vi "Sim_Main.vi"() -> ()   [LabVIEW 2009]
panel:
  in  "on or off":bool=TRUE
  in  "Right Thrust 2":dbl
  in  "Left Thrust 2":dbl
  out "Waveform Graph":cluster{dbl, "Delta t":dbl, "elements":dbl[]}(graph)
  in  "Inertia":dbl=10.0
  in  "max queue size (-1, unlimited)":i32=10
  out "XY Graph":T1(graph)
  in  "Mass":dbl=10.0
  in  "stop":bool
  in  "Delta t":dbl=0.01
  out "Time":dbl
  in  "Left Voltage":dbl
  in  "Right Voltage":dbl
  out "Right Thrust":dbl
  out "Left Thrust":dbl
  out "Theta":dbl
  out "Omega":dbl
  out "Alpha":dbl
  out "Ay":dbl
  out "Ax":dbl
  out "Vy":dbl
  out "Y":dbl
  out "Vx":dbl
  out "X":dbl
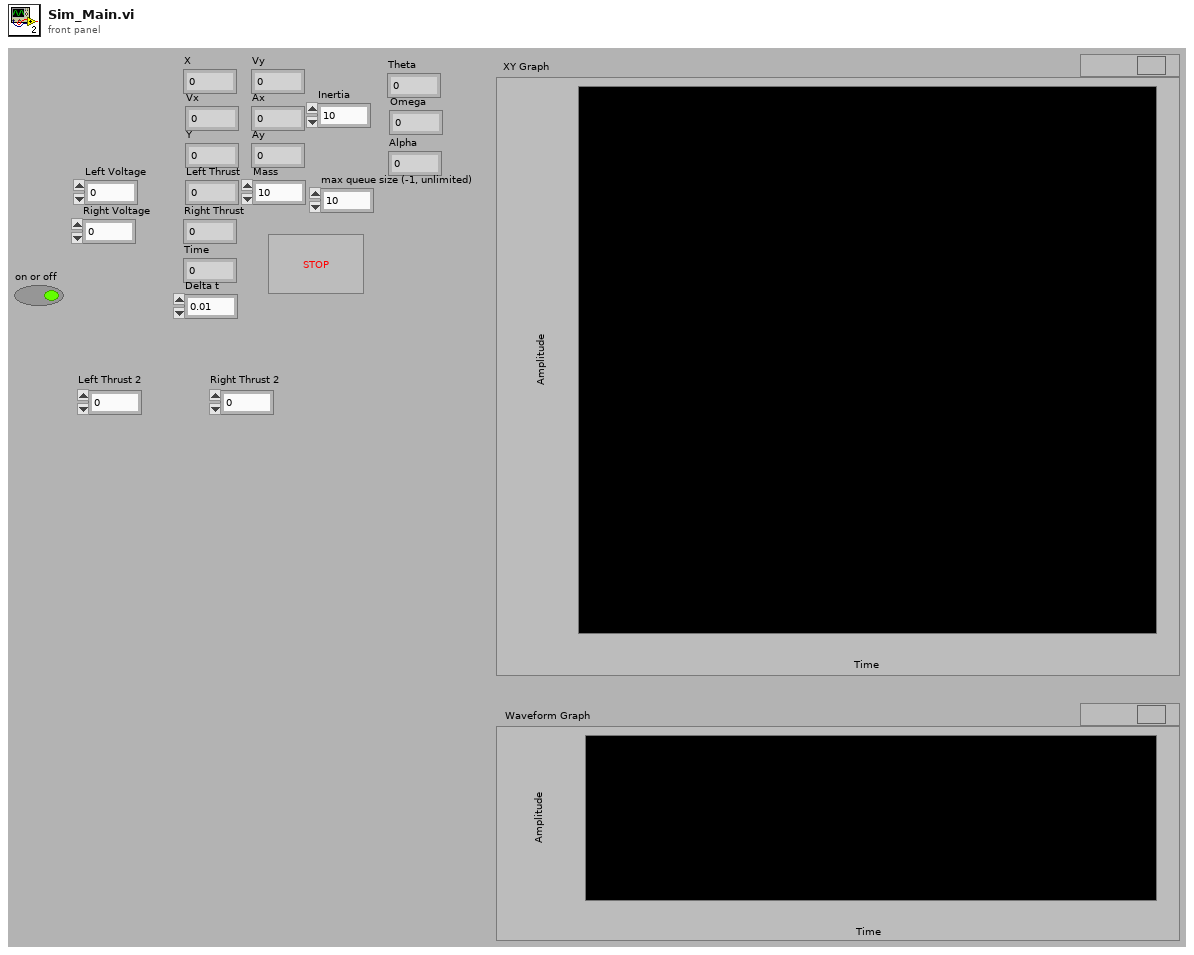
[diagram p1: front panel]
types:
  T1 = cluster{"initialized array":dbl[], "initialized array":dbl[]}[]
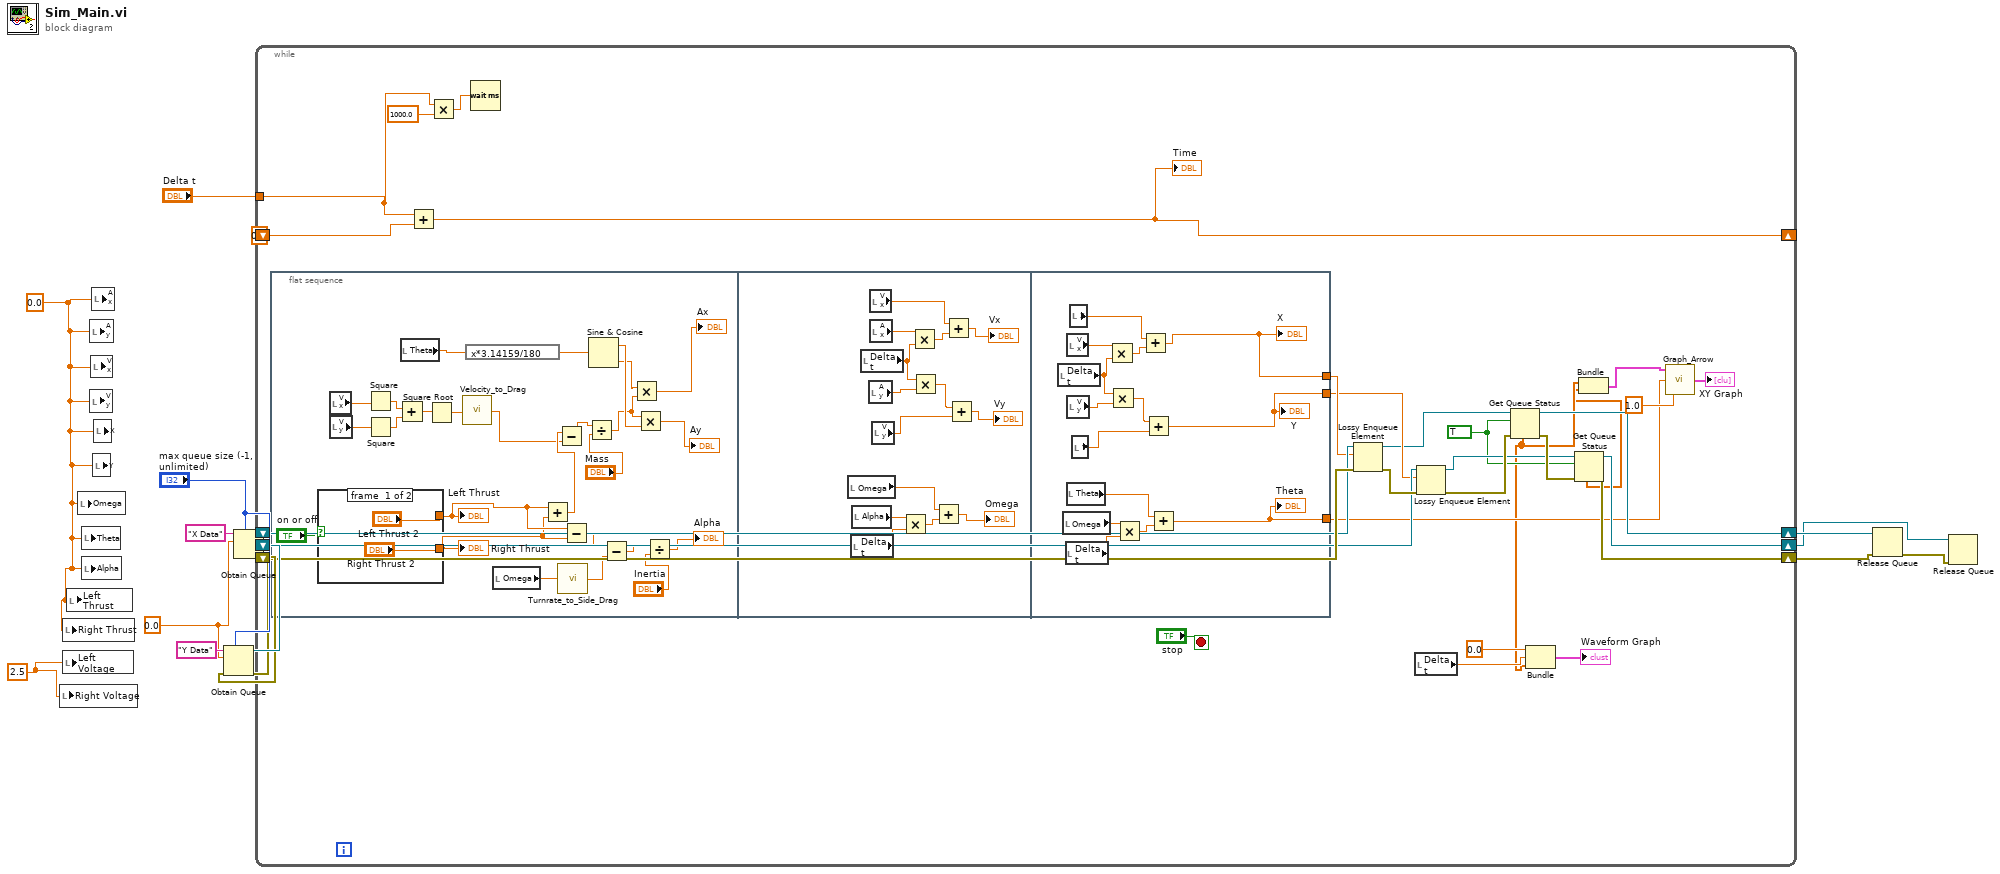
[diagram p0: block diagram]
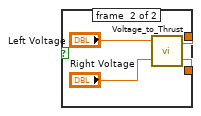
[diagram p2: hidden frame]
diagram:
  w1 = 2.5 ("Ax")
  w9 = 0.0 ("Ax")
  w2 = 0.0 ("Ax")
  n1 = local write "Right Voltage"(w1) -> ()
  n2 = local write "Right Thrust"(w2) -> ()
  n3 = local write "Left Voltage"(w1) -> ()
  n4 = local write "Left Thrust"(w2) -> ()
  n5 = local write "Omega"(w2) -> ()
  n6 = local write "Theta"(w2) -> ()
  n7 = local write "Alpha"(w2) -> ()
  n8 = local write "Ay"(w2) -> ()
  n9 = local write "Vy"(w2) -> ()
  n10 = local write "Vx"(w2) -> ()
  n11 = local write "Ax"(w2) -> ()
  n12 = local write "Y"(w2) -> ()
  n13 = local write "X"(w2) -> ()
  n14 = Obtain Queue(max queue size (-1, unlimited)="max queue size (-1, unlimited)", name (unnamed)="X Data", element data type=w9) -> (queue out=w11:refnum<queue>, error out=w8:errorcluster)  [unwired: 2 in, 1 out]
  n15 = Obtain Queue(max queue size (-1, unlimited)="max queue size (-1, unlimited)", name (unnamed)="Y Data", element data type=w9, error in (no error)=w8) -> (queue out=w10:refnum<queue>, error out=w7:errorcluster)  [unwired: 1 in, 1 out]
  n16 = while {
    tunnel: "Delta t" -> [w42]
    shift-right: [w43] -> _
    shift-left: 0.0 -> [w44]
    shift-right: [w26] -> w6
    shift-left: w11 -> [w36]
    shift-right: [w25] -> w4
    shift-left: w10 -> [w34]
    shift-right: [w24] -> w5
    shift-left: w7 -> [w37]
    stop <- "stop" stop-if-true
    w27 = TRUE ("return elements? (F)")
    n17 = flat-sequence {
      tunnel: [w98] -> w33
      tunnel: [w97] -> w32
      tunnel: [w92] -> w22
      frame #0 {
        n18 = case shown="False" "on or off" {
          tunnel: ["Left Thrust 2" w75] -> w62
          tunnel: ["Right Thrust 2" w74] -> w61
          frame #0 {
          }
          frame #1 {
            n19 = call "Voltage_to_Thrust.vi"("Right Voltage"="Right Voltage", "Left Voltage"="Left Voltage") -> ("Right Thrust"=w74:dbl, "Left Thrust"=w75:dbl)
          }
        }
        "Left Thrust" <- w62
        "Right Thrust" <- w61
        n20 = local read "Vx"() -> (w68:dbl)
        n21 = local read "Vy"() -> (w67:dbl)
        n22 = Square(x=w68) -> (x^2=w66:dbl)
        n23 = Square(x=w67) -> (x^2=w65:dbl)
        n24 = Add(x=w66, y=w65) -> (x+y=w64:dbl)
        n25 = local read "Theta"() -> (w71:dbl)
        n26 = Square Root(x=w64) -> (sqrt(x)=w63:dbl)
        n27 = call "Velocity_to_Drag.vi"("Velocity"=w63) -> ("Drag"=w59:dbl)
        n28 = expression code="x*3.14159/180"(w71) -> (w70:dbl)
        n29 = local read "Omega"() -> (w69:dbl)
        n30 = Add(x=w62, y=w61) -> (x+y=w60:dbl)
        n31 = Subtract(x=w60, y=w59) -> (x-y=w53:dbl)
        n32 = call "Turnrate_to_Side_Drag.vi"("Turn Rate"=w69) -> ("Side Drag"=w50:dbl)
        n33 = Subtract(x=w62, y=w61) -> (x-y=w51:dbl)
        n34 = Divide(x=w53, y="Mass") -> (x/y=w52:dbl)
        n35 = Sine & Cosine(0:w70) -> (1:w58:dbl, 2:w57:dbl)
        n36 = Subtract(x=w51, y=w50) -> (x-y=w49:dbl)
        n37 = Multiply(x=w57, y=w52) -> (x*y=→"Ax":dbl)
        n38 = Multiply(x=w52, y=w58) -> (x*y=→"Ay":dbl)
        n39 = Divide(x=w49, y="Inertia") -> (x/y=→"Alpha":dbl)
      }
      frame #1 {
        n40 = local read "Omega"() -> (w81:dbl)
        n41 = local read "Delta t"() -> (w82:dbl)
        n42 = local read "Alpha"() -> (w79:dbl)
        n43 = local read "Delta t"() -> (w87:dbl)
        n44 = local read "Ay"() -> (w88:dbl)
        n45 = local read "Vx"() -> (w89:dbl)
        n46 = local read "Ax"() -> (w91:dbl)
        n47 = local read "Vy"() -> (w85:dbl)
        n48 = Multiply(x=w79, y=w82) -> (x*y=w80:dbl)
        n49 = Multiply(x=w91, y=w87) -> (x*y=w90:dbl)
        n50 = Multiply(x=w87, y=w88) -> (x*y=w86:dbl)
        n51 = Add(x=w81, y=w80) -> (x+y=→"Omega":dbl)
        n52 = Add(x=w89, y=w90) -> (x+y=→"Vx":dbl)
        n53 = Add(x=w86, y=w85) -> (x+y=→"Vy":dbl)
      }
      frame #2 {
        n54 = local read "Delta t"() -> (w103:dbl)
        n55 = local read "Omega"() -> (w96:dbl)
        n56 = local read "Delta t"() -> (w93:dbl)
        n57 = local read "Theta"() -> (w94:dbl)
        n58 = local read "Vx"() -> (w99:dbl)
        n59 = local read "Vy"() -> (w102:dbl)
        n60 = local read "X"() -> (w101:dbl)
        n61 = local read "Y"() -> (w105:dbl)
        n62 = Multiply(x=w99, y=w103) -> (x*y=w100:dbl)
        n63 = Multiply(x=w103, y=w102) -> (x*y=w104:dbl)
        n64 = Multiply(x=w96, y=w93) -> (x*y=w95:dbl)
        n65 = Add(x=w101, y=w100) -> (x+y=w98:dbl)
        "X" <- w98
        n66 = Add(x=w104, y=w105) -> (x+y=w97:dbl)
        "Y" <- w97
        n67 = Add(x=w94, y=w95) -> (x+y=w92:dbl)
        "Theta" <- w92
      }
    }
    n68 = Add(x=w42, y=w44) -> (x+y=w43:dbl)
    "Time" <- w43
    n69 = Multiply(x=w42, y=1000.0) -> (x*y=w41:dbl)
    n70 = Wait (ms)(milliseconds to wait=w41) -> ()  [unwired: 1 out]
    n71 = Lossy Enqueue Element(queue=w36, element=w33, error in (no error)=w37) -> (queue out=w28:refnum<queue>, error out=w35:errorcluster)  [unwired: 2 out]
    n72 = local read "Delta t"() -> (w20:dbl)
    n73 = Lossy Enqueue Element(queue=w34, element=w32, error in (no error)=w35) -> (queue out=w29:refnum<queue>, error out=w30:errorcluster)  [unwired: 2 out]
    n74 = Get Queue Status(queue=w28, return elements? (F)=w27, error in (no error)=w30) -> (queue out=w26:refnum<queue>, error out=w31:errorcluster, elements=w19:dbl[])  [unwired: 5 out]
    n75 = Bundle(0.0, "Delta t"=w20, "elements"=w19) -> (→"Waveform Graph":cluster{dbl, "Delta t":dbl, "elements":dbl[]})  [unwired: 1 in]
    n76 = Get Queue Status(queue=w29, return elements? (F)=w27, error in (no error)=w31) -> (queue out=w25:refnum<queue>, error out=w24:errorcluster, elements=w18:dbl[])  [unwired: 5 out]
    n77 = Bundle("elements"=w19, "elements"=w18) -> (w23:cluster{"elements":dbl[], "elements":dbl[]})  [unwired: 1 in]
    n78 = call "Graph_Arrow.vi"("magnitude"=1.0, "Heading"=w22, "plot data"=w23) -> ("XY Graph"=→"XY Graph":T1)
  }
  n79 = Release Queue(queue=w6, error in (no error)=w5) -> (error out=w3:errorcluster)  [unwired: 1 in, 2 out]
  n80 = Release Queue(queue=w4, error in (no error)=w3) -> ()  [unwired: 1 in, 3 out]
